vi "FIXED FPGA ERRORS (PC).vi"() -> ()   [LabVIEW 2013]
uses:
  <vilib>/rvi/FXPMathLib/FxpDiv/subVIs/nifxpmath_Div_SimConfig.ctl
  <vilib>/rvi/FXPMathLib/FxpDiv/simVIs/DllFxpDivTemp_sub.vi
  <vilib>/rvi/FXPMathLib/FxpDiv/XNode/nifxpmath_Div.xnode
  <vilib>/rvi/FXPMathLib/FxpMul/XNode/nifxpmath_Multiplier.xnode
  <vilib>/rvi/FXPMathLib/FxpSub/XNode/nifxpmath_Sub.xnode
  <vilib>/rvi/FXPMathLib/FxpAdd/XNode/nifxpmath_Add.xnode
  <vilib>/rvi/FXPMathLib/sim/FxpSim.dll
panel:
  in  "NoiseAmpl":dbl
  in  "Pause":bool
  in  "sigLvl":dbl
  in  "milliseconds to wait":u32=100
  out "Waveform Chart 4":dbl(graph)
  out "Waveform Chart 2":dbl(graph)
  out "Waveform Chart 3":dbl(graph)
  out "Waveform Chart":dbl(graph)
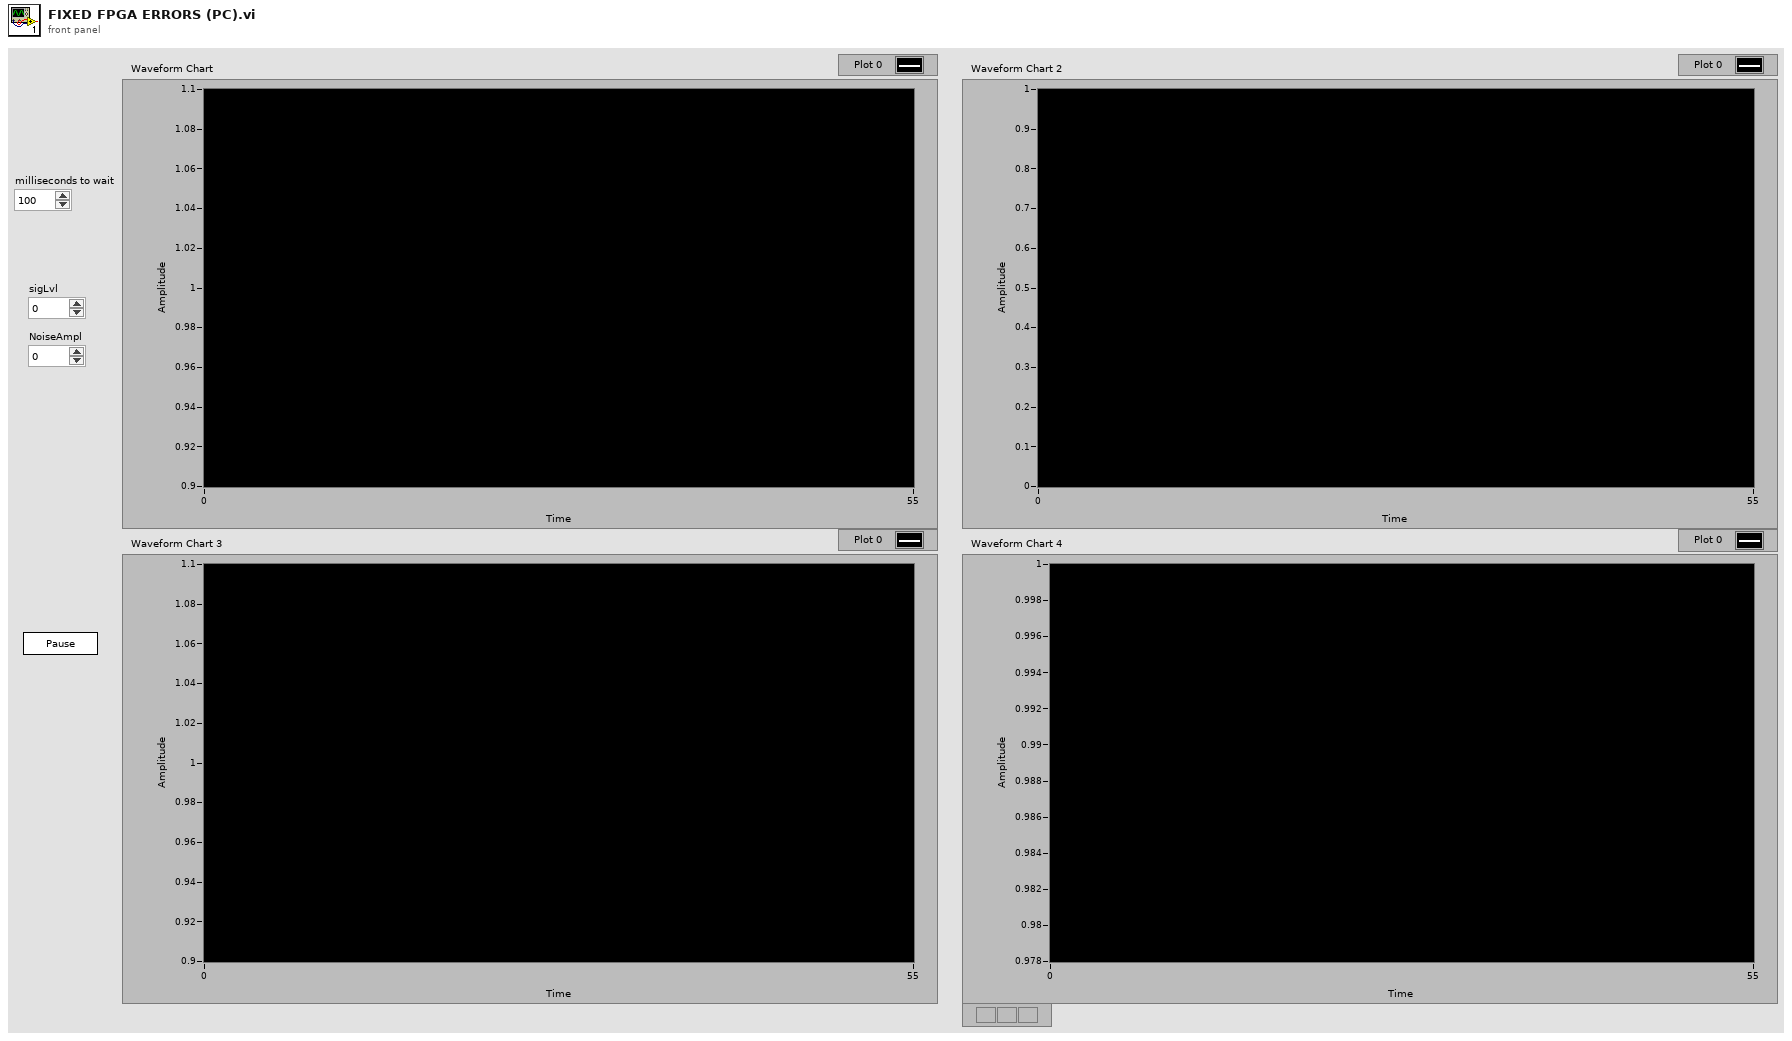
[diagram p1: front panel]
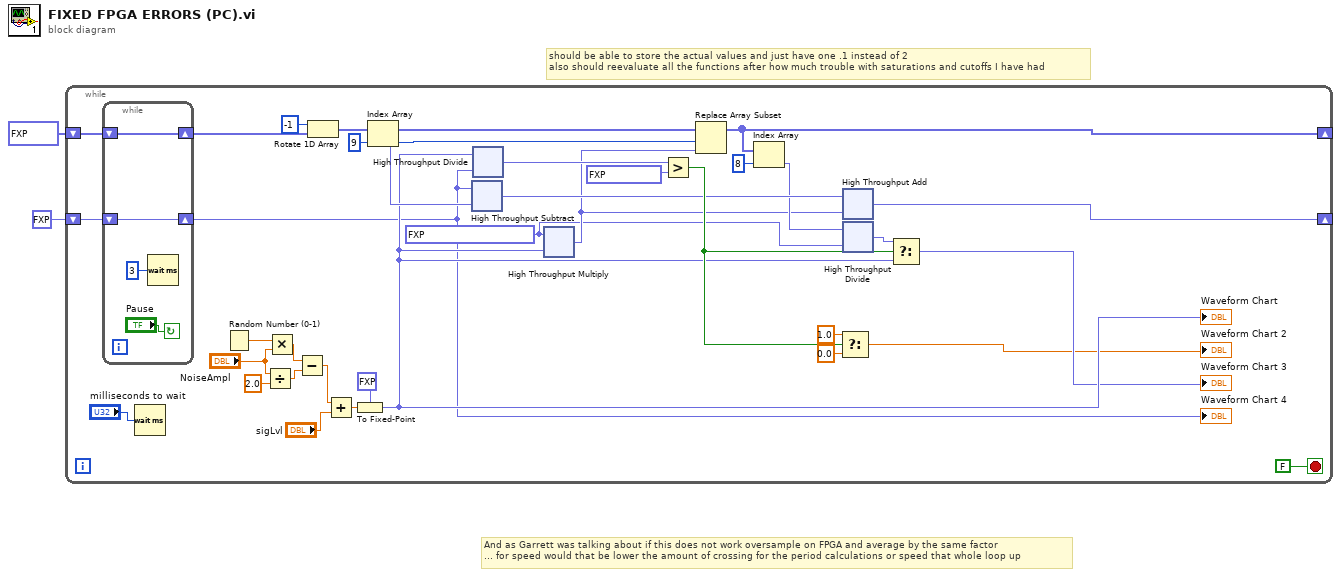
[diagram p0: block diagram]
diagram:
  # "And as Garrett was talking about if this does not work oversample on FPGA and average by the same factor\n... for speed would that be lower the amount of crossing for the period calculations or speed that whole loop up"
  # "should be able to store the actual values and just have one .1 instead of 2\nalso should reevaluate all the functions after how much trouble with saturations and cutoffs I have had"
  n1 = while {
    shift-right: [w36] -> _
    shift-left: fxp<+/-,32,16>[] [0.0, 0.0, 0.0, 0.0, 0.0, 0.0, 0.0, 0.0, 0.0, 0.0] -> [w28]
    shift-right: [w29] -> _
    shift-left: fxp<+/-,32,16> 0.0 ("x+y") -> [w27]
    stop <- FALSE stop-if-true
    w3 = fxp<+,24,5> 0.10000038146972656 ("x")
    w19 = 9 ("index")
    n2 = while {
      shift-right: [w95] -> w26
      shift-left: w28 -> [w95]
      shift-right: [w94] -> w7
      shift-left: w27 -> [w94]
      stop <- "Pause" continue-if-true
      n3 = Wait (ms)(milliseconds to wait=u32 3) -> ()  [unwired: 1 out]
    }
    "Waveform Chart 4" <- w7
    n4 = Wait (ms)(milliseconds to wait="milliseconds to wait") -> ()  [unwired: 1 out]
    n5 = Random Number (0-1)() -> (number: 0 to 1=w10:dbl)
    n6 = Divide(x="NoiseAmpl", y=2.0) -> (x/y=w13:dbl)
    n7 = Multiply(x=w10, y="NoiseAmpl") -> (x*y=w12:dbl)
    n8 = Subtract(x=w12, y=w13) -> (x-y=w11:dbl)
    n9 = Rotate 1D Array(1:w26, 2:-1 ("n")) -> (0:w23:fxp<+/-,32,16>[])
    n10 = Add(x=w11, y="sigLvl") -> (x+y=w25:dbl)
    n11 = To Fixed-Point(fixed-point type=fxp<+,32,16> 0.0 ("y"), number=w25) -> (fixed-point=w8:fxp<+,32,16>)
    "Waveform Chart" <- w8
    n12 = Index Array(array=w23, index=w19) -> (element=w22:fxp<+/-,32,16>)
    n13 = xnode "High Throughput Subtract"("x"=w7, "y"=w22) -> ("x-y"=w17:fxp<+/-,40,24>)
    n14 = xnode "High Throughput Divide"("x"=w8, "y"=w7) -> ("x/y"=w21:fxp<+/-,40,24>)
    n15 = xnode ("High Throughput Multiply")("x"=w3, "y"=w8) -> ("x*y"=w4:fxp<+,56,21>)
    n16 = Greater?(x=w21, y=fxp<+/-,34,24> 1.0302734375) -> (0:w31:bool)
    n17 = Replace Array Subset(array=w23, new element=w4, index=w19) -> (w36:fxp<+/-,32,16>[])
    n18 = Index Array(array=w36, index=8) -> (element=w16:fxp<+/-,32,16>)
    n19 = Select(t=1.0 ("Waveform Chart 3"), s=w31, f=0.0 ("Waveform Chart 3")) -> (s? t:f=→"Waveform Chart 2":dbl)
    n20 = xnode "High Throughput Add"("x"=w17, "y"=w4) -> ("x+y"=w29:fxp<+/-,60,25>)
    n21 = xnode "High Throughput Divide"("x"=w16, "y"=w3) -> ("x/y"=w15:fxp<+/-,40,24>)
    n22 = Select(t=w15, s=w31, f=w8) -> (s? t:f=→"Waveform Chart 3":fxp<+/-,40,24>)
  }
